vi "Read String.vi"(11 "String With Equals in":refnum<class "String With Equals.lvclass">) -> (2 "string":string, 3 "String With Equals out":refnum<class "String With Equals.lvclass">)   [LabVIEW 2023, in "String With Equals.lvclass"]
uses:
  String With Equals.lvclass
  String With Equals.lvclass/String With Equals.ctl
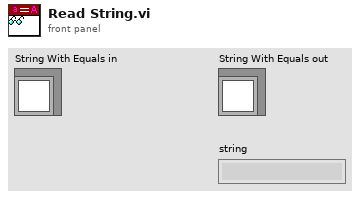
[diagram p1: front panel]
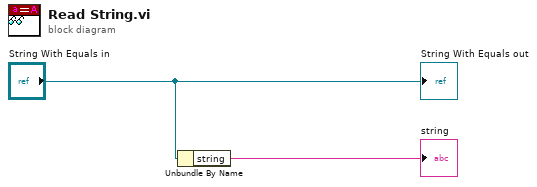
[diagram p0: block diagram]
diagram:
  n1 = Unbundle By Name("String With Equals in") -> ("string"=→"string":string)
  "String With Equals out" <- "String With Equals in"
